vi "CleanUp.vi"(0 "object in":refnum<class "Application.lvclass">, 5 "error in (no error)":errorcluster) -> (14 "object out":refnum<class "Application.lvclass">, 19 "error out":errorcluster)   [LabVIEW 2024, in "Application.lvclass"]
uses:
  Application.lvclass
  Application.lvclass/Application.ctl
  AD2_SDK_class/AD2_SDK.lvclass
  Prior_Zmotor_class/Prior_Zmotor.lvclass
  CetoniPump_class/CetoniPump.lvclass
  Hamamatsu_class/Hamamatsu.lvclass
  Valve_class/Valve.lvclass
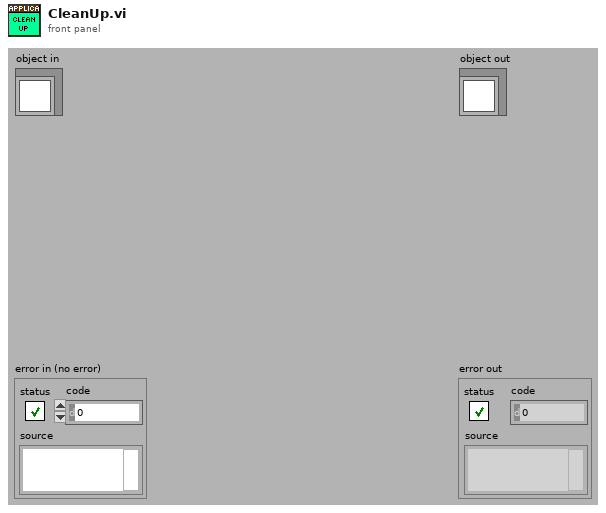
[diagram p1: front panel]
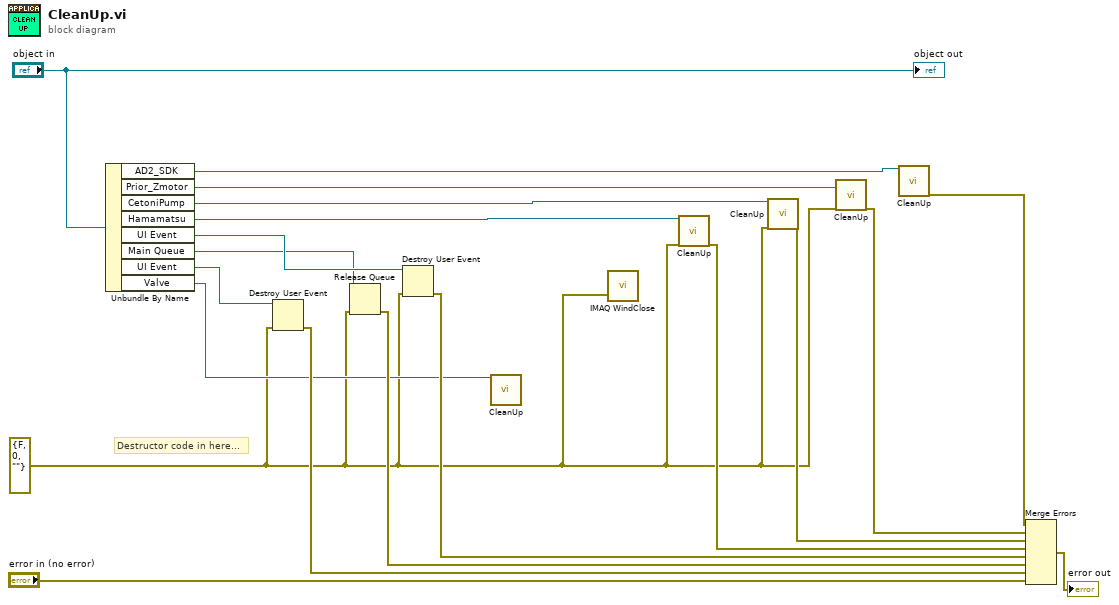
[diagram p0: block diagram]
diagram:
  w5 = errorcluster {"status"=FALSE, "code"=0, "source"=""} ("error in (no error)")
  # "Destructor code in here..."
  n1 = Unbundle By Name("object in") -> ("AD2_SDK"=w2:refnum<class "AD2_SDK.lvclass">, "Prior_Zmotor"=w4:refnum<class "Prior_Zmotor.lvclass">, "CetoniPump"=w7:refnum<class "CetoniPump.lvclass">, "Hamamatsu"=w10:refnum<class "Hamamatsu.lvclass">, "UI Event"=w17:refnum<user-event>, "Main Queue"=w16:refnum<queue>, "UI Event"=w15:refnum<user-event>, "Valve"=w8:refnum<class "Valve.lvclass">)
  n2 = Destroy User Event(user event=w15, error in=w5) -> (error out=w12:errorcluster)
  n3 = Release Queue(queue=w16, error in (no error)=w5) -> (error out=w13:errorcluster)  [unwired: 1 in, 2 out]
  n4 = Destroy User Event(user event=w17, error in=w5) -> (error out=w14:errorcluster)
  n5 = call-dynamic "CleanUp.vi"("object in"=w8) -> ()  [unwired: 17 in, 2 out]
  n6 = call "IMAQ WindClose"("error in (no error)"=w5) -> ()  [unwired: 5 in, 1 out]
  n7 = call-dynamic "CleanUp.vi"("object in"=w10, "error in (no error)"=w5) -> ("error out"=w9:errorcluster)  [unwired: 16 in, 1 out]
  n8 = call-dynamic "CleanUp.vi"("object in"=w7, "error in (no error)"=w5) -> ("error out"=w6:errorcluster)  [unwired: 16 in, 1 out]
  n9 = call-dynamic "CleanUp.vi"("object in"=w4, "error in (no error)"=w5) -> ("error out"=w3:errorcluster)  [unwired: 16 in, 1 out]
  n10 = call-dynamic "CleanUp.vi"("object in"=w2) -> ("error out"=w1:errorcluster)  [unwired: 17 in, 1 out]
  n11 = Merge Errors(w1, w3, w6, w9, w14, w13, w12, "error in (no error)") -> (→"error out":errorcluster)
  "object out" <- "object in"
